vi "Test Find and ID Instruments.vi"() -> ()   [LabVIEW 2016]
uses:
  Device/Device type.ctl
  <vilib>/Instr/_visa.llb/VISA Find Search Mode.ctl
panel:
  in  "Search Mode":T1 items=["Canonical Names Only"=0, "Aliases Only"=2, "Include Matching Aliases"=3, "Include All Aliases"=4]
  out "ID":T2[](array[typedef])
  out "Found":bool[](array[boolean])
  out "find list":string[](array[string])
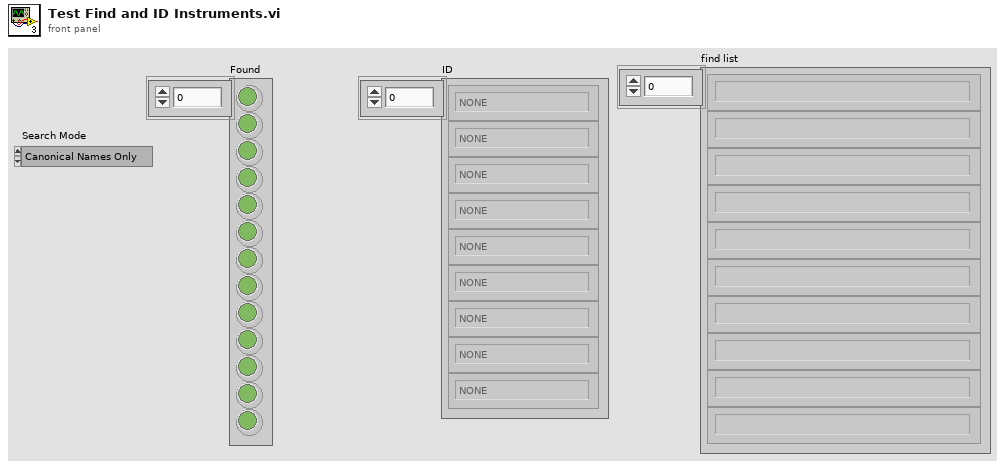
[diagram p1: front panel]
types:
  T1 = typedef "VISA Find Search Mode.ctl" = u32
  T2 = typedef "Device type.ctl" = enum16{"NONE", "Neocera 21", "LakeShore 335", "LakeShore 336", "LakeShore 340", "LkShr 340 chA&B", "LakeShore 370", "SRS 850", "SRS 830", "LR 700", "EG&G 5302", "EG&G 7260", "EG&G 7280", "AH 2500", "Keithley meter", "Keithley electrometer", "Keithley 182", "HP 5385", "HP 53181", "HP 53132", "ITC503", "IPS120", "Oxford Mercury IPS", "Oxford PS", "Test", "DC Facility Magnet", "Cryomagnetics PS", "Keithley 2400", "Keithley current source", "Cryo-Con 22C", "HP87NN", "HP4395A", "Agilent 34410A"}
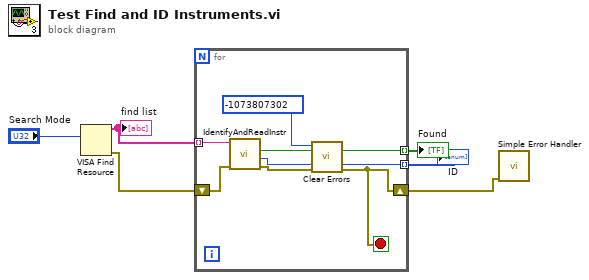
[diagram p0: block diagram]
diagram:
  n1 = VISA Find Resource(10:"Search Mode") -> (0:w5:errorcluster, 3:w6:string[])  [unwired: 2 in, 1 out]
  "find list" <- w6
  n2 = for {
    tunnel: w6 -> [w13] mode=indexing
    tunnel: [w12] -> w3 mode=indexing
    tunnel: [w11] -> w2 mode=indexing
    shift-right: [w8] -> w4
    shift-left: w5 -> [w10]
    stop <- w8 stop-if-true
    n3 = call "IdentifyAndReadInstr.vi"("error in (no error)"=w10, "VISA Resource Name"=w13) -> ("error out"=w9:errorcluster, "Instrument"=w11:T2, "Identified"=w12:bool)  [unwired: 6 in, 1 out]
    n4 = call <vilib>:"Clear Errors.vi"("error in (no error)"=w9, "specific error code to clear (0: all)"=-1073807302) -> ("error out"=w8:errorcluster)  [unwired: 4 in, 1 out]
  }
  "Found" <- w3
  "ID" <- w2
  n5 = call <vilib>:"Simple Error Handler.vi"("error in (no error)"=w4) -> ()  [unwired: 4 in, 5 out]
